vi "Create.vi"(10 "Info":T1[](array[typedef])) -> (3 "ConfigMonitorInfoValue out":refnum<class "ConfigMonitorInfoValue.lvclass">)   [LabVIEW 2020, in "Volatus.lvlib" / "ConfigMonitorInfoValue.lvclass"]
uses:
  ConfigMonitorInfoValue.lvclass
  ConfigMonitorInfoValue.lvclass/ConfigMonitorInfoValue.ctl
  Config Alert Module/Node Config Info.ctl
  Config Alert Module/Config Monitor Module.lvclass
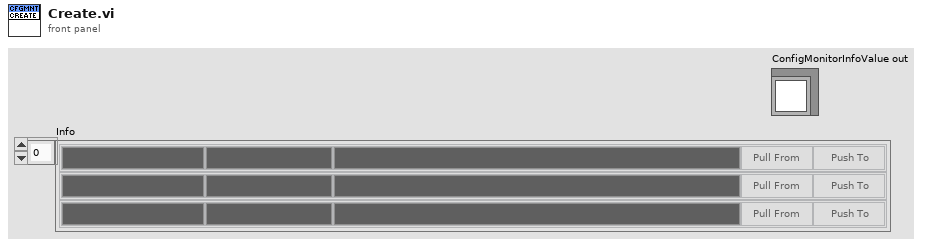
[diagram p1: front panel]
types:
  T1 = typedef "Volatus.lvlib/Config Monitor Module.lvclass/Node Config Info.ctl" = cluster{"Node":string, "Config Version":string, "Config Hash":string, "Pull":bool, "Push":bool, "Version Color":u32, "Hash Color":u32, "Node Color":u32}
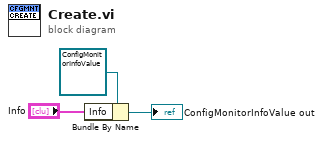
[diagram p0: block diagram]
diagram:
  n1 = Bundle By Name(cluster=refnum<class "ConfigMonitorInfoValue.lvclass"> refnum ("ConfigMonitorInfoValue in"), "Info"="Info") -> (→"ConfigMonitorInfoValue out":refnum<class "ConfigMonitorInfoValue.lvclass">)
